vi "Builder-ext.vi"(8 "error in (no error)":errorcluster, 11 "Builder":refnum<class "Builder.lvclass">) -> (0 "error out":errorcluster, 1 "Library Description":string, 2 "Built PPL Path":path)   [LabVIEW 2019]
uses:
  Builder/Builder.lvclass
panel:
  in  "View Project Files":bool
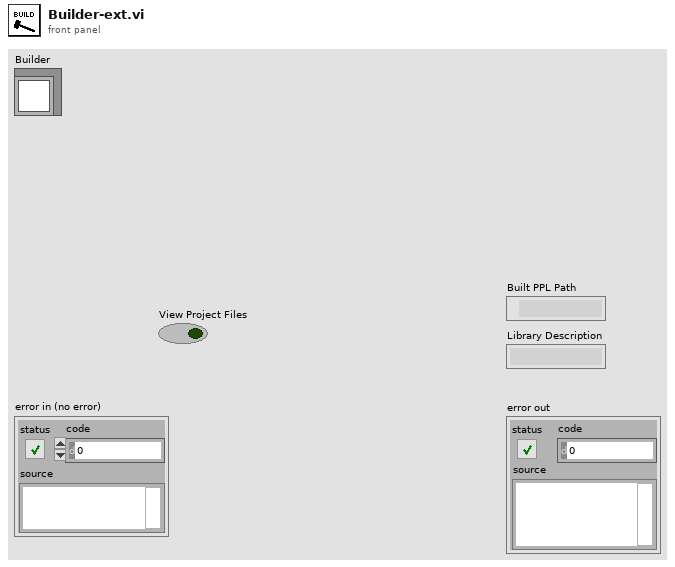
[diagram p1: front panel]
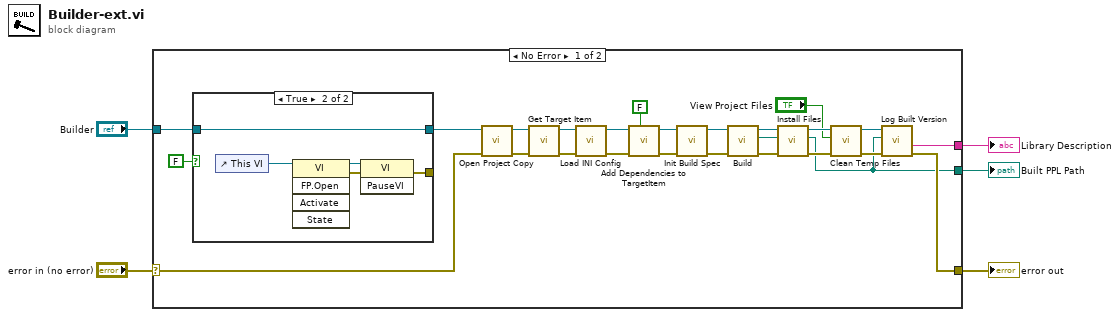
[diagram p0: block diagram]
diagram:
  n1 = case shown="No Error" "error in (no error)" {
    selector: "error in (no error)" -> [w16 w38]
    tunnel: [w10 w38] -> w5
    tunnel: "Builder" -> [w17 _]
    tunnel: [w8 _] -> w2
    tunnel: [w6 _] -> w1
    frame No Error {
      n2 = case shown="True" FALSE {
        tunnel: [_ w34] -> _
        tunnel: w17 -> [w32 w33]
        tunnel: [w32 w33] -> w15
        frame False {
        }
        frame True {
          n3 = control-ref of="This VI"() -> (w37:refnum<vi>)
          n4 = invoke class="VI" method="FP.Open"(reference=w37) -> (reference out=w36:refnum<vi>, error out=w35:errorcluster)  [unwired: 4 in, 3 out]
          n5 = invoke class="VI" method="PauseVI"(reference=w36, error in=w35) -> (error out=w34:errorcluster)  [unwired: 1 in, 2 out]
        }
      }
      n6 = call "Open Project Copy.vi"("error in"=w16, "Builder in"=w15) -> ("error out"=w31:errorcluster, "Builder out"=w29:refnum<class "Builder.lvclass">)  [unwired: 8 in]
      n7 = call "Get Target Item.vi"("error in (no error)"=w31, "Builder in"=w29) -> ("error out"=w30:errorcluster, "Builder out"=w27:refnum<class "Builder.lvclass">)  [unwired: 8 in]
      n8 = call "Load INI Config.vi"("error in (no error)"=w30, "Builder in"=w27) -> ("error out"=w24:errorcluster, "Builder out"=w25:refnum<class "Builder.lvclass">)  [unwired: 8 in]
      n9 = call "Add Dependencies to TargetItem.vi"("Add to Project"=FALSE, "error in (no error)"=w24, "Builder in"=w25) -> ("error out"=w22:errorcluster, "Builder out"=w23:refnum<class "Builder.lvclass">)  [unwired: 7 in]
      n10 = call "Init Build Spec.vi"("error in (no error)"=w22, "Builder in"=w23) -> ("error out"=w20:errorcluster, "Builder out"=w21:refnum<class "Builder.lvclass">)  [unwired: 7 in, 1 out]
      n11 = call "Build.vi"("error in (no error)"=w20, "Builder in"=w21) -> ("error out"=w19:errorcluster, "Built PPL Path"=w7:path, "Builder out"=w18:refnum<class "Builder.lvclass">)  [unwired: 7 in]
      n12 = call "Install Files.vi"("error in (no error)"=w19, "Generated PPL"=w7, "Builder in"=w18) -> ("error out"=w12:errorcluster, "PPL Path"=w6:path, "Builder out"=w14:refnum<class "Builder.lvclass">)  [unwired: 6 in]
      n13 = call "Clean Temp Files.vi"("error in (no error)"=w12, "Retain Project?"="View Project Files", "Builder in"=w14) -> ("error out"=w11:errorcluster, "Builder out"=w9:refnum<class "Builder.lvclass">)  [unwired: 7 in]
      n14 = call "Log Built Version.vi"("error in (no error)"=w11, "Generated PPL"=w6, "Builder in"=w9) -> ("error out"=w10:errorcluster, "Library Description"=w8:string)  [unwired: 6 in, 1 out]
    }
    frame Error {
    }
  }
  "error out" <- w5
  "Library Description" <- w2
  "Built PPL Path" <- w1
